vi "Scan DQMH Modules and create Maps.vi"(7 "Progress bar":refnum<vi>, 8 "error in":errorcluster, 9 "Include Dependencies":bool, 10 "Target Selection":string, 11 "Project":string) -> (0 "error out":errorcluster, 1 "Tree Map out":T1, 2 "map ref out":map{string, refnum<vi>}(c390), 3 "DQMH Modules Info":T2)   [LabVIEW 2019, in "Panther Dashboard.lvlib"]
doc: "Gets the Singleton and Cloneable references and creates a list of each type of DQMH Modules"
uses:
  Panther Dashboard.lvlib
  DQMH Modules Info--cluster.ctl
  Module type--enum.ctl
  Project References--cluster.ctl
  <vilib>/National Instruments/Tree Map/Tree Map Data.ctl
  <vilib>/National Instruments/Tree Map/Tree Map.lvlib
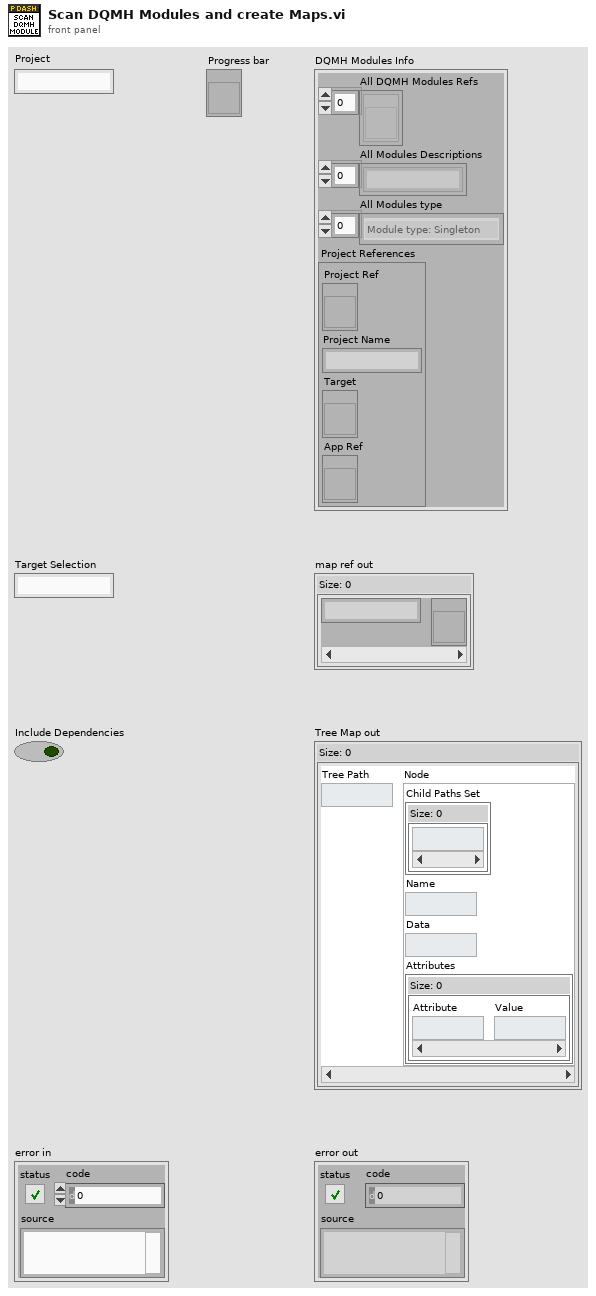
[diagram p1: front panel]
types:
  T1 = typedef "Tree Map.lvlib/Tree Map Data.ctl" = map{string, cluster{"Child Paths Set":set{string}, "Name":string, "Data":string, "Attributes":map{string, string}}}
  T2 = typedef "Panther Dashboard.lvlib/DQMH Modules Info--cluster.ctl" = cluster{"All DQMH Modules Refs":refnum<vi>[], "All Modules Descriptions":string[], "All Modules type":T3[], "Project References":T4}
  T3 = typedef "Panther Dashboard.lvlib/Module type--enum.ctl" = enum16{"Module type: Singleton", "Module type: Cloneable"}
  T4 = typedef "Panther Dashboard.lvlib/Project References--cluster.ctl" = cluster{"Project Ref":refnum<vi>, "Project Name":string, "Target":refnum<vi>, "App Ref":refnum<vi>}
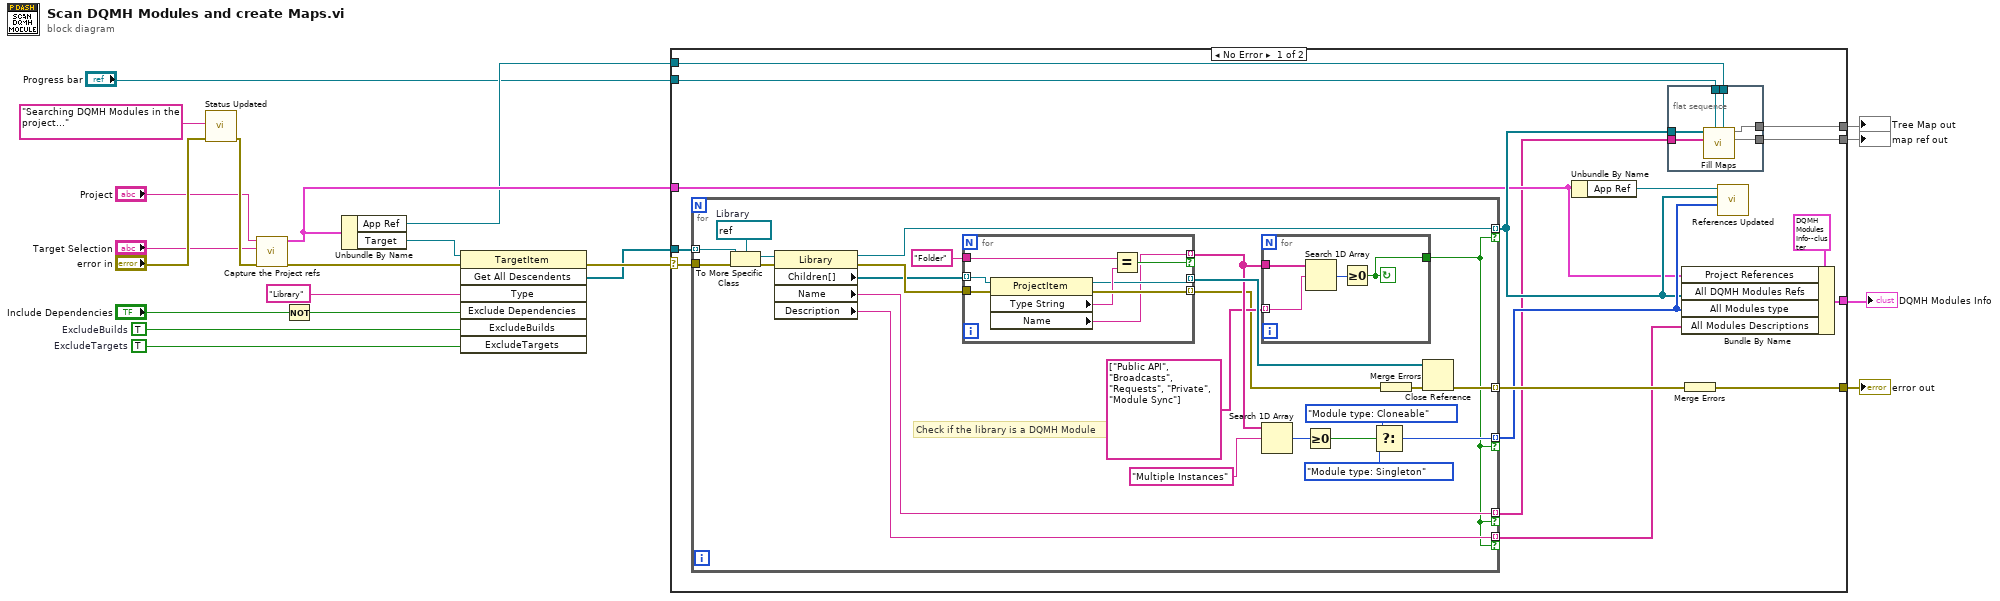
[diagram p0: block diagram]
diagram:
  w15 = TRUE  # ExcludeTargets
  w16 = TRUE  # ExcludeBuilds
  n1 = call "Status Updated.vi"("error in (no error)"="error in", "Status"="Searching DQMH Modules in the project...") -> ("error out"=w17:errorcluster)  [unwired: 9 in]
  n2 = call "Capture the Project refs.vi"("error in"=w17, "Target Selection"="Target Selection", "Project Selection"="Project") -> ("error out"=w20:errorcluster, "References"=w7:T4)  [unwired: 7 in]
  n3 = Not(x="Include Dependencies") -> (.not. x?=w11:bool)
  n4 = Unbundle By Name(w7) -> ("App Ref"=w5:refnum<vi>, "Target"=w6:refnum<vi>)
  n5 = invoke class="TargetItem" method="Get All Descendents"(reference=w6, error in=w20, "Type"="Library", "Exclude Dependencies"=w11, "ExcludeBuilds"=w16, "ExcludeTargets"=w15) -> (error out=w19:errorcluster, "All Descendents"=w8:refnum<vi>[])  [unwired: 1 in, 5 out]
  n6 = case shown="No Error" w19 {
    selector: w19 -> [w37 w80]
    tunnel: [w36 w80] -> w21
    tunnel: [w33 _] -> w12
    tunnel: w8 -> [w30 _]
    tunnel: [w32 _] -> w10
    tunnel: [w31 _] -> w9
    tunnel: w7 -> [w27 _]
    tunnel: w5 -> [w23 _]
    tunnel: "Progress bar" -> [w22 _]
    frame No Error {
      n7 = for {
        tunnel: [w49] -> w28 mode=indexing if=w44
        tunnel: w30 -> [w62] mode=indexing
        tunnel: [w67] -> w35 mode=indexing
        tunnel: w37 -> [w64]
        tunnel: [w61] -> w29 mode=indexing if=w44
        tunnel: [w46] -> w25 mode=indexing if=w44
        tunnel: [w45] -> w24 mode=indexing if=w44
        w47 = refnum<vi> refnum  # Library
        # "Check if the library is a DQMH Module"
        n8 = To More Specific Class(target class=w47, reference=w62, error in=w64) -> (specific class reference=w48:refnum<vi>, error out=w63:errorcluster)
        n9 = property class="Library"(reference=w48, error in=w63) -> (reference out=w49:refnum<vi>, error out=w66:errorcluster, "Children[]"=w59:refnum<vi>[], "Name"=w45:string, "Description"=w46:string)
        n10 = for {
          tunnel: [w72] -> w55 mode=indexing if=w73
          tunnel: w66 -> [w79]
          tunnel: [w78] -> w53 mode=indexing
          tunnel: [w75] -> w58 mode=indexing
          tunnel: w59 -> [w77] mode=indexing
          tunnel: "Folder" ("Type") -> [w74]
          n11 = property class="ProjectItem"(reference=w77, error in=w79) -> (reference out=w75:refnum<vi>, error out=w78:errorcluster, "Type String"=w76:string, "Name"=w72:string)
          n12 = Equal?(x=w74, y=w76) -> (x = y?=w73:bool)
        }
        n13 = for {
          tunnel: string[] ["Public API", "Broadcasts", "Requests", "Private", "Module Sync"] -> [w71] mode=indexing
          tunnel: w55 -> [w70]
          tunnel: [w68] -> w44
          stop <- w68 continue-if-true
          n14 = Search 1D Array(1D array=w70, element=w71) -> (index of element=w69:i32)  [unwired: 1 in]
          n15 = Greater Or Equal To 0?(x=w69) -> (x >= 0?=w68:bool)
        }
        n16 = Search 1D Array(1D array=w55, element="Multiple Instances") -> (index of element=w57:i32)  [unwired: 1 in]
        n17 = Greater Or Equal To 0?(x=w57) -> (x >= 0?=w52:bool)
        n18 = Select(t=Module_type--enum."Module type: Cloneable", s=w52, f=Module_type--enum."Module type: Singleton" ("Module type")) -> (s? t:f=w61:T3)
        n19 = Merge Errors(w53) -> (w65:errorcluster)
        n20 = Close Reference(reference=w58, error in (no error)=w65) -> (error out=w67:errorcluster)
      }
      n21 = Unbundle By Name(w27) -> ("App Ref"=w26:refnum<vi>)
      n22 = flat-sequence {
        tunnel: [w43] -> w32
        tunnel: [w42] -> w31
        tunnel: w28 -> [w41]
        tunnel: w24 -> [w40]
        tunnel: w22 -> [w38]
        tunnel: w23 -> [w39]
        frame #0 {
          n23 = call "Fill Maps.vi"("App Ref"=w39, "Progress bar"=w38, "Module names"=w40, "DQMH Modules"=w41) -> ("map ref out"=w43:map{string, refnum<vi>}, "Tree Map out"=w42:T1)  [unwired: 6 in]
        }
      }
      n24 = Bundle By Name(cluster=T2 {"All DQMH Modules Refs"=[], "All Modules Descriptions"=[], "All Modules type"=[], "Project References"={"Project Ref"=refnum, "Project Name"="", "Target"=refnum, "App Ref"=refnum}} ("DQMH Modules Info"), "Project References"=w27, "All DQMH Modules Refs"=w28, "All Modules type"=w29, "All Modules Descriptions"=w25) -> (w33:T2)
      n25 = Merge Errors(w35) -> (w36:errorcluster)
      n26 = call "References Updated.vi"("Modules Types"=w29, "Modules"=w28, "Application Instance"=w26) -> ()  [unwired: 8 in, 1 out]
    }
    frame Error {
    }
  }
  "error out" <- w21
  "DQMH Modules Info" <- w12
  "map ref out" <- w10
  "Tree Map out" <- w9
